vi "mathArcadeDrive.vi"(9 "Range":dbl, 10 "Wheel":dbl, 11 "Throttle":cluster{"Left":dbl, "Right":dbl}) -> (3 "Drive":cluster{"Left":dbl, "Right":dbl})   [LabVIEW 2011]
panel:
  # "Basically adds and subtracts Wheel from Throttle, used in auto."
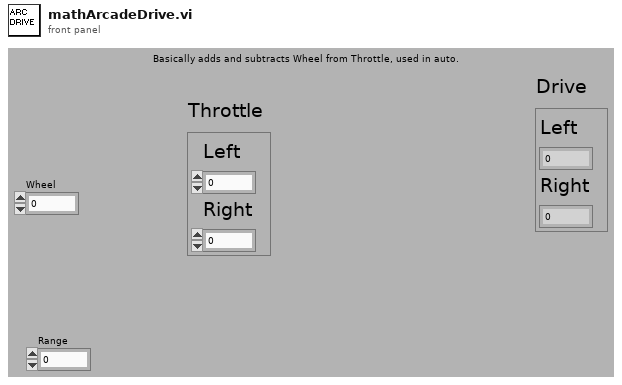
[diagram p1: front panel]
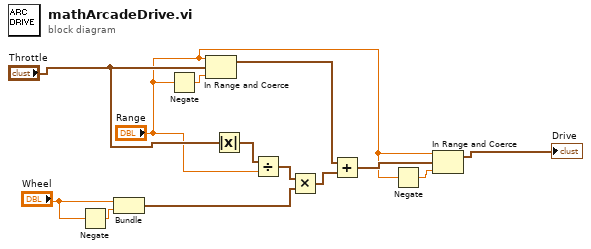
[diagram p0: block diagram]
diagram:
  n1 = Negate(x="Wheel") -> (-x=w9:dbl)
  n2 = Bundle("Wheel"="Wheel", w9) -> (w2:cluster{"Wheel":dbl, dbl})  [unwired: 1 out]
  n3 = Negate(x="Range") -> (-x=w13:dbl)
  n4 = In Range and Coerce(upper limit="Range", x="Throttle", lower limit=w13) -> (coerced(x)=w7:cluster{"Left":dbl, "Right":dbl})  [unwired: 1 out]
  n5 = Absolute Value(x="Throttle") -> (abs(x)=w5:cluster{"Left":dbl, "Right":dbl})
  n6 = Divide(x=w5, y="Range") -> (x/y=w3:cluster{"Left":dbl, "Right":dbl})
  n7 = Multiply(x=w3, y=w2) -> (x*y=w1:cluster{dbl, dbl})
  n8 = Add(x=w7, y=w1) -> (x+y=w8:cluster{dbl, dbl})
  n9 = Negate(x="Range") -> (-x=w12:dbl)
  n10 = In Range and Coerce(upper limit="Range", x=w8, lower limit=w12) -> (coerced(x)=→"Drive":cluster{dbl, dbl})  [unwired: 1 out]
